vi "Errors FGV.vi"(6 "Function":enum16{"Put", "Create", "Get"}(ring), 8 "Get error":errorcluster) -> (0 "Error Out":errorcluster)   [LabVIEW 2020, in "Error Handler.lvlib"]
uses:
  Error Handler.lvlib
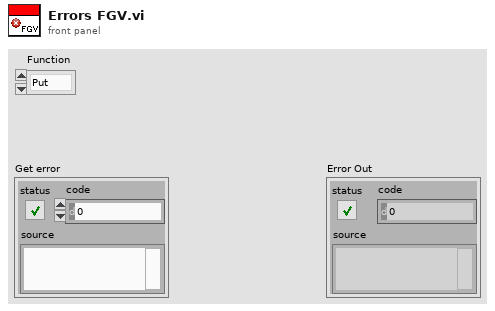
[diagram p1: front panel]
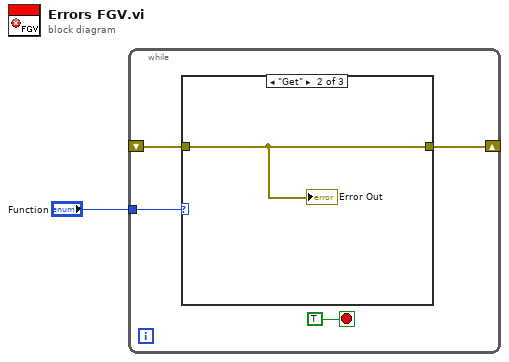
[diagram p0: block diagram]
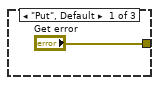
[diagram p2: hidden frame]
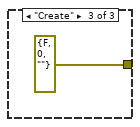
[diagram p3: hidden frame]
diagram:
  n1 = while {
    tunnel: "Function" -> [w4]
    shift-right: [w2] -> _
    shift-left: _ -> [w3]
    stop <- TRUE stop-if-true
    n2 = case shown="\"Get\"" w4 {
      tunnel: w3 -> [_ w7 _]
      tunnel: ["Get error" w7 errorcluster {"status"=FALSE, "code"=0, "source"=""} ("Get error")] -> w2
      frame "Put", Default {
      }
      frame "Get" {
        "Error Out" <- w7
      }
      frame "Create" {
      }
    }
  }
